vi "Findmidpoints-Toolingpinsutility.vi"(8 "2D Array of Error":dbl[][](array[numeric]), 9 "2D Array of Data":dbl[][](array[numeric]), 10 "Number of points to considet for the mid point":dbl=2.0, 11 "Sample Size":i32=3) -> (2 "Std Devs":dbl[][](array[numeric]), 3 "Averages":dbl[][](array[numeric]))   [LabVIEW 2016]
uses:
  <vilib>/Analysis/NI_AALBase.lvlib
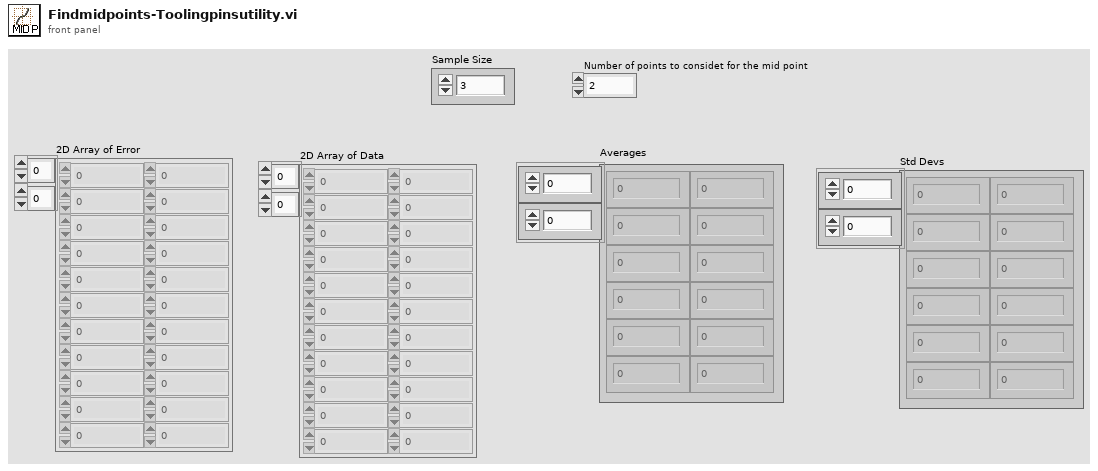
[diagram p1: front panel]
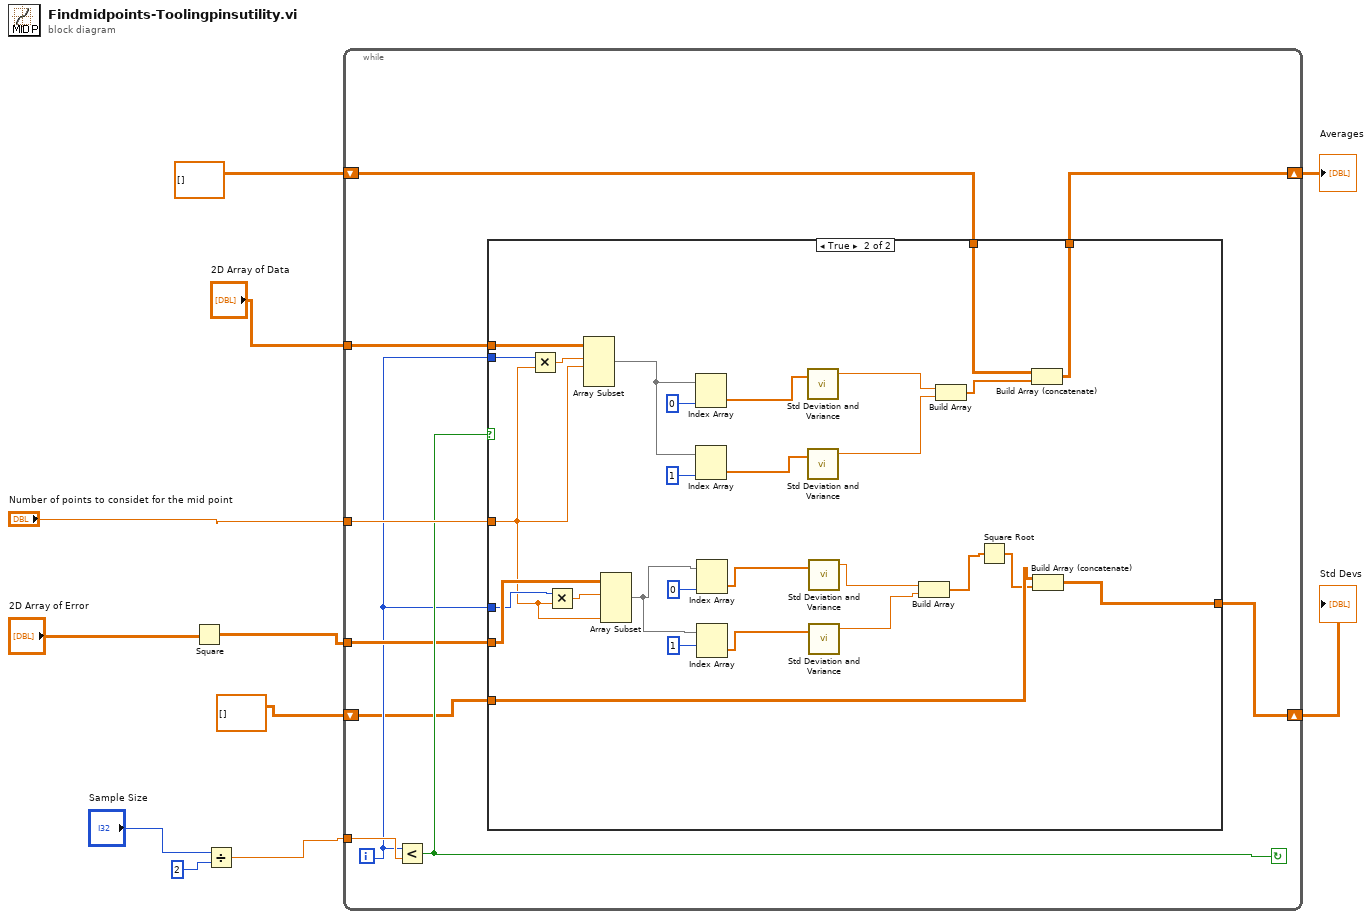
[diagram p0: block diagram]
diagram:
  n1 = Square(x="2D Array of Error") -> (x^2=w3:dbl[][])
  n2 = Divide(x="Sample Size", y=2) -> (x/y=w6:dbl)
  n3 = while {
    tunnel: w6 -> [w21]
    tunnel: "2D Array of Data" -> [w20]
    tunnel: "Number of points to considet for the mid point" -> [w19]
    shift-right: [w17] -> w9
    shift-left: dbl[][] [] -> [w18]
    tunnel: w3 -> [w15]
    shift-right: [w13] -> w2
    shift-left: dbl[][] [] -> [w12]
    i -> [w14]
    stop <- w16 continue-if-true
    n4 = Less?(x=w14, y=w21) -> (x < y?=w16:bool)
    n5 = case shown="True" w16 {
      tunnel: w20 -> [_ w51]
      tunnel: w14 -> [_ w49]
      tunnel: w19 -> [_ w32]
      tunnel: w18 -> [w23 w40]
      tunnel: [w23 w39] -> w17
      tunnel: [w22 w38] -> w13
      tunnel: w15 -> [_ w34]
      tunnel: w14 -> [_ w33]
      tunnel: w12 -> [w22 w26]
      frame False {
      }
      frame True {
        n6 = Multiply(x=w49, y=w32) -> (x*y=w50:dbl)
        n7 = Multiply(x=w33, y=w32) -> (x*y=w35:dbl)
        n8 = Array Subset(array=w51, index (row)=w50, length (row)=w32) -> (w46:dbl[][])  [unwired: 2 in]
        n9 = Array Subset(array=w34, index (row)=w35, length (col)=w32) -> (w31:dbl[][])  [unwired: 2 in]
        n10 = Index Array(array=w46, index (col)=0 ("disabled index (col)")) -> (element=w45:dbl[])  [unwired: 1 in]
        n11 = Index Array(array=w46, index (col)=1 ("disabled index (col)")) -> (element=w44:dbl[])  [unwired: 1 in]
        n12 = Index Array(array=w31, index (col)=0) -> (element=w30:dbl[])  [unwired: 1 in]
        n13 = Index Array(array=w31, index (row)=1) -> (element=w29:dbl[])  [unwired: 1 in]
        n14 = call <vilib>:"Std Deviation and Variance.vi"("X"=w45) -> ("mean"=w43:dbl)  [unwired: 1 in, 2 out]
        n15 = call <vilib>:"Std Deviation and Variance.vi"("X"=w44) -> ("mean"=w42:dbl)  [unwired: 1 in, 2 out]
        n16 = call <vilib>:"Std Deviation and Variance.vi"("X"=w30) -> ("mean"=w28:dbl)  [unwired: 1 in, 2 out]
        n17 = call <vilib>:"Std Deviation and Variance.vi"("X"=w29) -> ("mean"=w27:dbl)  [unwired: 1 in, 2 out]
        n18 = Build Array(w28, w27) -> (w25:dbl[])
        n19 = Build Array(w43, w42) -> (w41:dbl[])
        n20 = Square Root(x=w25) -> (sqrt(x)=w24:dbl[])
        n21 = Build Array (concatenate)(w40, w41) -> (w39:dbl[][])
        n22 = Build Array (concatenate)(w26, w24) -> (w38:dbl[][])
      }
    }
  }
  "Averages" <- w9
  "Std Devs" <- w2
